vi "Information.vi"(8 "error in (no error)":errorcluster, 9 "Context":T1, 10 "Information":refnum<class "Information.lvclass">, 11 "Combined Measurement in":refnum<class "Combined Measurement.lvclass">) -> (0 "error out":errorcluster, 3 "Combined Measurement out":refnum<class "Combined Measurement.lvclass">)   [LabVIEW 2021, in "Combined Measurement.lvclass"]
uses:
  Combined Measurement.lvclass
  Publish-Subscribe/Interfaces/Information/Information.lvclass
  Publish-Subscribe/Context.ctl
  NHMFL_Core/Libraries/Instruments/Results/Acquired Result/Acquired Result.lvclass
  Measurements/Response Synchronizer/Response Synchronizer.lvclass
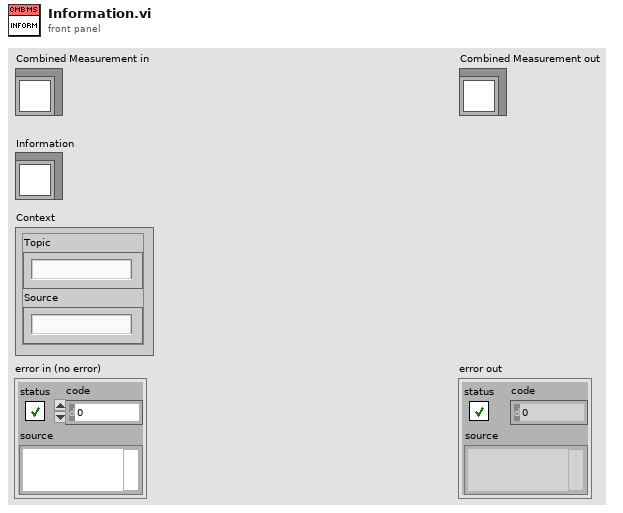
[diagram p1: front panel]
types:
  T1 = typedef "Context.ctl" = cluster{"Topic":string, "Source":string}
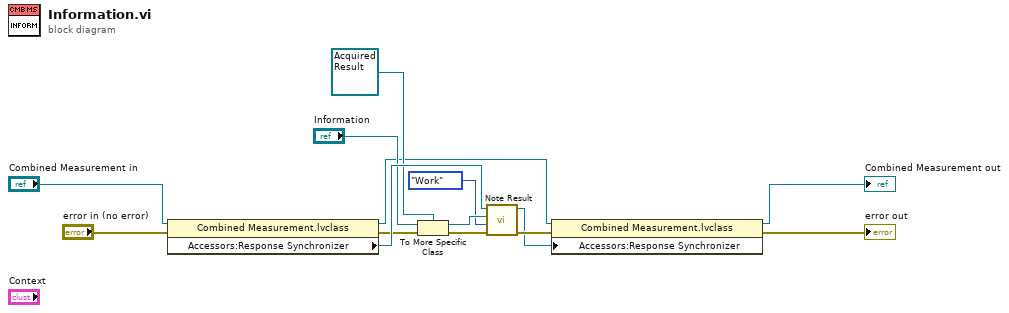
[diagram p0: block diagram]
diagram:
  n1 = property class="Combined Measurement.lvclass"(reference="Combined Measurement in", error in="error in (no error)") -> (reference out=w4:refnum<class "Combined Measurement.lvclass">, error out=w8:errorcluster, "Accessors:Response Synchronizer"=w13:refnum<class "Response Synchronizer.lvclass">)
  n2 = To More Specific Class(target class=refnum<class "Acquired Result.lvclass"> refnum ("Acquired Result.lvclass"), reference="Information", error in=w8) -> (specific class reference=w12:refnum<class "Acquired Result.lvclass">, error out=w7:errorcluster)
  n3 = call-dynamic "Note Result.vi"("error in (no error)"=w7, "Stage"=enum16{"Init", "Work"}."Work", "Acquired Result.lvclass"=w12, "Response Synchronizer in"=w13) -> ("error out"=w5:errorcluster, "Response Synchronizer out"=w2:refnum<class "Response Synchronizer.lvclass">)  [unwired: 4 in, 2 out]
  n4 = property class="Combined Measurement.lvclass"(reference=w4, error in=w5, "Accessors:Response Synchronizer"=w2) -> (reference out=→"Combined Measurement out":refnum<class "Combined Measurement.lvclass">, error out=→"error out":errorcluster)
